vi "Stop.vi"(8 "Error In":errorcluster) -> (0 "Error Out":errorcluster)   [LabVIEW 2014, in "Logger.lvlib"]
uses:
  Logger.lvlib
  Private/_Control Action.ctl
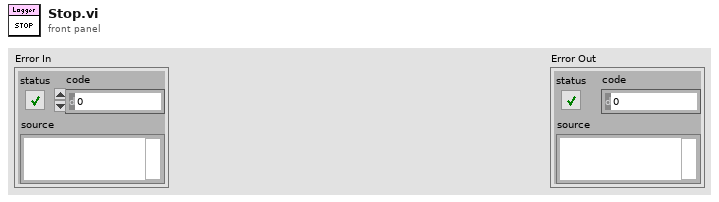
[diagram p1: front panel]
types:
  T1 = typedef "Logger.lvlib/_Control Action.ctl" = enum16{"Initialize", "Get", "Set", "Shutdown"}
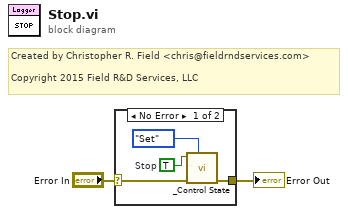
[diagram p0: block diagram]
diagram:
  # "Created by Christopher R. Field <chris@fieldrndservices.com>\n\nCopyright 2015 Field R&D Services, LLC"
  n1 = case shown="No Error" "Error In" {
    selector: "Error In" -> [w4 w7]
    tunnel: [w3 w7] -> w1
    frame No Error {
      w5 = TRUE  # Stop
      n2 = call "_Control State.vi"("Action"=_Control_Action."Set", "Error In"=w4, "Set Value"=w5) -> ("Error Out"=w3:errorcluster)  [unwired: 7 in, 1 out]
    }
    frame Error {
    }
  }
  "Error Out" <- w1
